vi "KE6221 -- Set Sine Wave Params.vi"(0 "Resource In":refnum<visa-resource-name>, 1 "Check For SCPI Errors? (T)":bool=TRUE, 7 "Sine Wave Params In":T1={"Frequency (Hz)"=1000.0, "Amplitude (A)"=0.001, "Offset (A)"=0.0, "Ranging Mode"=enum."Best", "Fixed Range"=enum."2mA", "Playback Mode"=enum."Time", "Time (s)"=1.0, "Num Cycles"=1.0, "Phase\nMarker?"=FALSE, "Phase Marker (deg)"=180.0, "Trig Link Line"=enum."1"} {"Offset (A)" min=-0.105 max=0.105 format="%.4p"; "Num Cycles" min=0.001 max=99999999900.0 format="%.3p"; "Time (s)" min=1e-07 max=999999.999 format="%.3p"; "Phase Marker (deg)" min=0.0 max=360.0 format="%.3f"; "Amplitude (A)" min=2e-12 max=0.105 format="%.3p"; "Frequency (Hz)" min=0.001 max=100000.0 format="%.3p"}, 11 "error in (no error)":errorcluster, 12 "Read Back Set Values? (T)":bool=TRUE) -> (4 "Resource Out (dupl)":refnum<visa-resource-name>, 8 "Sine Wave Params Out":T1={"Frequency (Hz)"=1000.0, "Amplitude (A)"=0.001, "Offset (A)"=0.0, "Ranging Mode"=enum."Best", "Fixed Range"=enum."2mA", "Playback Mode"=enum."Time", "Time (s)"=1.0, "Num Cycles"=1.0, "Phase\nMarker?"=FALSE, "Phase Marker (deg)"=180.0, "Trig Link Line"=enum."1"} {"Offset (A)" min=-0.105 max=0.105 format="%.4p"; "Num Cycles" min=0.001 max=99999999900.0 format="%.3p"; "Time (s)" min=1e-07 max=999999.999 format="%.3p"; "Phase Marker (deg)" min=0.0 max=360.0 format="%.3f"; "Amplitude (A)" min=2e-12 max=0.105 format="%.3p"; "Frequency (Hz)" min=0.001 max=100000.0 format="%.3p"}, 15 "error out":errorcluster)   [LabVIEW 2019, in "Keithley 622x.lvlib"]
doc: "Sets the parameters for a sine wave. Note that this VI can only be used with the 6221, since the 6220 doesn't support this feature."
uses:
  Keithley 622x.lvlib
  Typedefs/KE6221 -- Wave Sine Wave Params.ctl
  Low Level/Typedefs/KE6221 -- Wave Frequency.ctl
  Low Level/Typedefs/KE6221 -- Wave Amplitude.ctl
  Source/Typedefs/KE622x -- Current Level.ctl
  Low Level/Typedefs/KE6221 -- Wave Ranging Mode.ctl
  Source/Typedefs/KE622x -- Current Ranges.ctl
  Low Level/Typedefs/KE6221 -- Wave Playback Mode.ctl
  Low Level/Typedefs/KE6221 -- Wave Playback Time.ctl
  Low Level/Typedefs/KE6221 -- Wave Playback Num Cycles.ctl
  Low Level/Typedefs/KE6221 -- Wave Phase Marker.ctl
  Trigger/Low Level/Typedefs/KE622x -- Trig Link Line.ctl
  Low Level/Typedefs/KE6221 -- Wave Type.ctl
  Source/Typedefs/KE622x -- Current Range.ctl
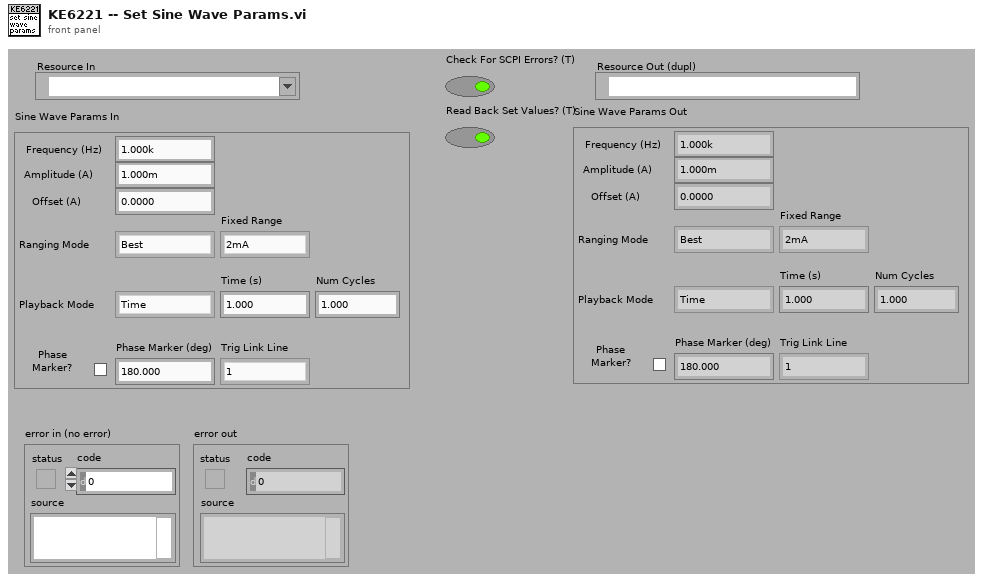
[diagram p1: front panel]
types:
  T1 = typedef "Keithley 622x.lvlib/KE6221 -- Wave Sine Wave Params.ctl" = cluster{"Frequency (Hz)":T2, "Amplitude (A)":T3, "Offset (A)":T4, "Ranging Mode":T5, "Fixed Range":T6, "Playback Mode":T7, "Time (s)":T8, "Num Cycles":T9, "Phase\nMarker?":bool, "Phase Marker (deg)":T10, "Trig Link Line":T11}
  T2 = typedef "Keithley 622x.lvlib/KE6221 -- Wave Frequency.ctl" = dbl
  T3 = typedef "Keithley 622x.lvlib/KE6221 -- Wave Amplitude.ctl" = dbl
  T4 = typedef "Keithley 622x.lvlib/KE622x -- Current Level.ctl" = dbl
  T5 = typedef "Keithley 622x.lvlib/KE6221 -- Wave Ranging Mode.ctl" = enum16{"Best", "Fixed"}
  T6 = typedef "Keithley 622x.lvlib/KE622x -- Current Ranges.ctl" = enum16{"2nA", "20nA", "200nA", "2uA", "20uA", "200uA", "2mA", "20mA", "100mA"}
  T7 = typedef "Keithley 622x.lvlib/KE6221 -- Wave Playback Mode.ctl" = enum16{"Time", "Num Cycles"}
  T8 = typedef "Keithley 622x.lvlib/KE6221 -- Wave Playback Time.ctl" = dbl
  T9 = typedef "Keithley 622x.lvlib/KE6221 -- Wave Playback Num Cycles.ctl" = dbl
  T10 = typedef "Keithley 622x.lvlib/KE6221 -- Wave Phase Marker.ctl" = dbl
  T11 = typedef "Keithley 622x.lvlib/KE622x -- Trig Link Line.ctl" = enum16{"1", "2", "3", "4", "5", "6"}
  T12 = typedef "Keithley 622x.lvlib/KE6221 -- Wave Type.ctl" = enum16{"Sinusoid", "Square", "Ramp", "Arbitrary 0", "Arbitrary 1", "Arbitrary 2", "Arbitrary 3", "Arbitrary 4"}
  T13 = typedef "Keithley 622x.lvlib/KE622x -- Current Range.ctl" = cluster{"Auto Range?":bool, "Man / Selected\nRange":T6}
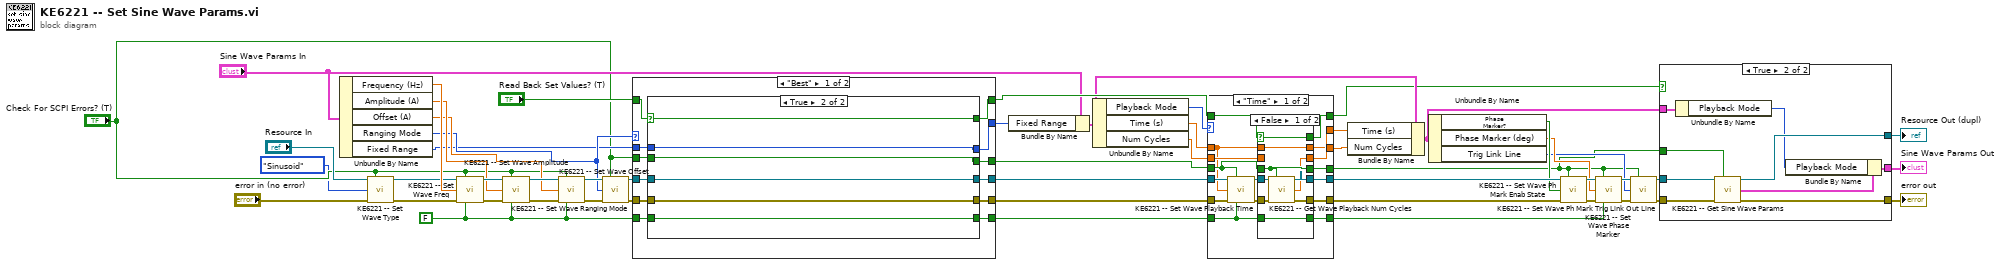
[diagram p0: block diagram]
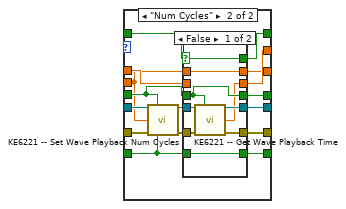
[diagram p4: hidden frame]
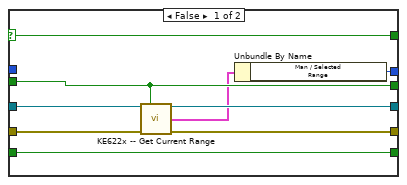
[diagram p6: hidden frame]
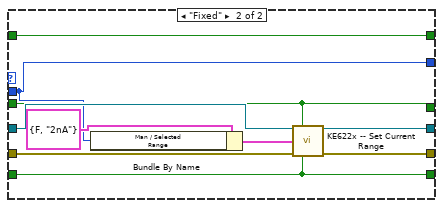
[diagram p7: hidden frame]
diagram:
  w17 = FALSE
  n1 = Unbundle By Name("Sine Wave Params In") -> ("Frequency (Hz)"=w40:T2, "Amplitude (A)"=w39:T3, "Offset (A)"=w38:T4, "Ranging Mode"=w37:T5, "Fixed Range"=w36:T6)
  n2 = call "KE6221 -- Set Wave Type.vi"("Resource In"="Resource In", "Check For SCPI Errors? (T)"="Check For SCPI Errors? (T)", "Wave Type"=KE6221_--_Wave_Type."Sinusoid", "error in (no error)"="error in (no error)") -> ("Resource Out (dupl)"=w8:refnum<visa-resource-name>, "error out"=w7:errorcluster)  [unwired: 10 in]
  n3 = call "KE6221 -- Set Wave Freq.vi"("Resource In"=w8, "Check For SCPI Errors? (T)"="Check For SCPI Errors? (T)", "Wave Frequency In (Hz)"=w40, "error in (no error)"=w7, "Read Back Set Value? (T)"=w17) -> ("Resource Out (dupl)"=w52:refnum<visa-resource-name>, "error out"=w51:errorcluster)  [unwired: 8 in, 1 out]
  n4 = call "KE6221 -- Set Wave Amplitude.vi"("Resource In"=w52, "Check For SCPI Errors? (T)"="Check For SCPI Errors? (T)", "Wave Amplitude In"=w39, "error in (no error)"=w51, "Read Back Set Value? (T)"=w17) -> ("Resource Out (dupl)"=w48:refnum<visa-resource-name>, "error out"=w47:errorcluster)  [unwired: 8 in, 1 out]
  n5 = call "KE6221 -- Set Wave Offset.vi"("Resource In"=w48, "Check For SCPI Errors? (T)"="Check For SCPI Errors? (T)", "Wave Offset In (A)"=w38, "error in (no error)"=w47, "Read Back Set Value? (T)"=w17) -> ("Resource Out (dupl)"=w46:refnum<visa-resource-name>, "error out"=w45:errorcluster)  [unwired: 8 in, 1 out]
  n6 = call "KE6221 -- Set Wave Ranging Mode.vi"("Resource In"=w46, "Check For SCPI Errors? (T)"="Check For SCPI Errors? (T)", "Ranging Mode"=w37, "error in (no error)"=w45) -> ("Resource Out (dupl)"=w50:refnum<visa-resource-name>, "error out"=w49:errorcluster)  [unwired: 10 in]
  n7 = case shown="\"Best\"" w37 {
    tunnel: w50 -> [w63 w89]
    tunnel: w49 -> [w62 w88]
    tunnel: [w59 w87] -> w33
    tunnel: [w60 w86] -> w30
    tunnel: "Check For SCPI Errors? (T)" -> [w61 w82]
    tunnel: w36 -> [w56 w81]
    tunnel: "Read Back Set Values? (T)" -> [w64 w83]
    tunnel: [w58 w82] -> w29
    tunnel: [w57 w83] -> w28
    tunnel: [w55 w81] -> w26
    tunnel: w17 -> [w54 w80]
    tunnel: [w53 w80] -> w16
    frame "Best" {
      n8 = case shown="True" w64 {
        selector: w64 -> [w68 w79]
        tunnel: w63 -> [w73 w77]
        tunnel: w62 -> [w72 w76]
        tunnel: w61 -> [w69 w78]
        tunnel: [w71 w76] -> w60
        tunnel: [w70 w77] -> w59
        tunnel: [w69 w78] -> w58
        tunnel: [w68 w79] -> w57
        tunnel: w56 -> [_ w75]
        tunnel: [w66 w75] -> w55
        tunnel: w54 -> [w65 w74]
        tunnel: [w65 w74] -> w53
        frame False {
          n9 = call "KE622x -- Get Current Range.vi"("Resource In"=w73, "Check For SCPI Errors? (T)"=w69, "error in (no error)"=w72) -> ("Resource Out (dupl)"=w70:refnum<visa-resource-name>, "Current Range"=w67:T13, "error out"=w71:errorcluster)  [unwired: 10 in]
          n10 = Unbundle By Name(w67) -> ("Man / Selected\nRange"=w66:T6)
        }
        frame True {
        }
      }
    }
    frame "Fixed" {
      n11 = Bundle By Name(cluster=T13 {"Auto Range?"=FALSE, "Man / Selected\nRange"=enum."2nA"} ("Current Range In"), "Man / Selected\nRange"=w81) -> (w84:T13)
      n12 = call "KE622x -- Set Current Range.vi"("Resource In"=w89, "Check For SCPI Errors? (T)"=w82, "Current Range In"=w84, "error in (no error)"=w88, "Read Back Set Values? (T)"=w80) -> ("Resource Out (dupl)"=w87:refnum<visa-resource-name>, "error out"=w86:errorcluster)  [unwired: 8 in, 1 out]
    }
  }
  n13 = Bundle By Name(cluster="Sine Wave Params In", "Fixed Range"=w26) -> (w25:T1)
  n14 = Unbundle By Name(w25) -> ("Playback Mode"=w34:T7, "Time (s)"=w32:T8, "Num Cycles"=w31:T9)
  n15 = case shown="\"Time\"" w34 {
    tunnel: w33 -> [w105 w137]
    tunnel: w32 -> [w94 w128]
    tunnel: w31 -> [w96 w126]
    tunnel: w30 -> [w104 w136]
    tunnel: w29 -> [w100 w132]
    tunnel: w28 -> [w103 w135]
    tunnel: [w95 w125] -> w23
    tunnel: [w99 w131] -> w11
    tunnel: [w98 w130] -> w22
    tunnel: [w97 w129] -> w21
    tunnel: [w93 w127] -> w24
    tunnel: w16 -> [w92 w124]
    tunnel: [w91 w123] -> w15
    tunnel: [w90 w122] -> w14
    frame "Time" {
      n16 = call "KE6221 -- Set Wave Playback Time.vi"("Resource In"=w105, "Check For SCPI Errors? (T)"=w100, "Playback Time (s) In"=w94, "error in (no error)"=w104, "Read Back Set Value? (T)"=w92) -> ("Resource Out (dupl)"=w102:refnum<visa-resource-name>, "error out"=w101:errorcluster)  [unwired: 8 in, 1 out]
      n17 = case shown="False" w103 {
        selector: w103 -> [w106 w115]
        tunnel: w102 -> [w114 w119]
        tunnel: w101 -> [w113 w120]
        tunnel: w100 -> [w112 w121]
        tunnel: [w112 w121] -> w99
        tunnel: [w111 w120] -> w97
        tunnel: [w110 w119] -> w98
        tunnel: w96 -> [_ w118]
        tunnel: [w109 w118] -> w95
        tunnel: w94 -> [w108 w117]
        tunnel: [w108 w117] -> w93
        tunnel: w92 -> [w107 w116]
        tunnel: [w107 w116] -> w91
        tunnel: [w106 w115] -> w90
        frame False {
          n18 = call "KE6221 -- Get Wave Playback Num Cycles.vi"("Resource In"=w114, "Check For SCPI Errors? (T)"=w112, "error in (no error)"=w113) -> ("Resource Out (dupl)"=w110:refnum<visa-resource-name>, "Num Cycles"=w109:T9, "error out"=w111:errorcluster)  [unwired: 10 in]
        }
        frame True {
        }
      }
    }
    frame "Num Cycles" {
      n19 = call "KE6221 -- Set Wave Playback Num Cycles.vi"("Resource In"=w137, "Check For SCPI Errors? (T)"=w132, "Num Cycles In"=w126, "error in (no error)"=w136, "Read Back Set Value? (T)"=w124) -> ("Resource Out (dupl)"=w134:refnum<visa-resource-name>, "error out"=w133:errorcluster)  [unwired: 8 in, 1 out]
      n20 = case shown="False" w135 {
        selector: w135 -> [w138 w147]
        tunnel: w134 -> [w146 w151]
        tunnel: w133 -> [w145 w152]
        tunnel: w132 -> [w144 w153]
        tunnel: [w144 w153] -> w131
        tunnel: [w143 w152] -> w129
        tunnel: [w142 w151] -> w130
        tunnel: w128 -> [_ w150]
        tunnel: [w141 w150] -> w127
        tunnel: w126 -> [w140 w149]
        tunnel: [w140 w149] -> w125
        tunnel: w124 -> [w139 w148]
        tunnel: [w139 w148] -> w123
        tunnel: [w138 w147] -> w122
        frame False {
          n21 = call "KE6221 -- Get Wave Playback Time.vi"("Resource In"=w146, "Check For SCPI Errors? (T)"=w144, "error in (no error)"=w145) -> ("Resource Out (dupl)"=w142:refnum<visa-resource-name>, "Playback Time (s)"=w141:T8, "error out"=w143:errorcluster)  [unwired: 10 in]
        }
        frame True {
        }
      }
    }
  }
  n22 = Bundle By Name(cluster=w25, "Time (s)"=w24, "Num Cycles"=w23) -> (w10:T1)
  n23 = Unbundle By Name(w10) -> ("Phase\nMarker?"=w20:bool, "Phase Marker (deg)"=w19:T10, "Trig Link Line"=w18:T11)
  n24 = call "KE6221 -- Set Wave Ph Mark Enab State.vi"("Resource In"=w22, "Check For SCPI Errors? (T)"=w11, "Phase Marker Enabled?"=w20, "error in (no error)"=w21) -> ("Resource Out (dupl)"=w44:refnum<visa-resource-name>, "error out"=w43:errorcluster)  [unwired: 10 in]
  n25 = call "KE6221 -- Set Wave Phase Marker.vi"("Resource In"=w44, "Check For SCPI Errors? (T)"=w11, "Phase Marker In (deg)"=w19, "error in (no error)"=w43, "Read Back Set Value? (T)"=w15) -> ("Resource Out (dupl)"=w42:refnum<visa-resource-name>, "error out"=w41:errorcluster)  [unwired: 8 in, 1 out]
  n26 = call "KE6221 -- Set Wave Ph Mark Trig Link Out Line.vi"("Resource In"=w42, "Check For SCPI Errors? (T)"=w11, "Trig Link Out Line"=w18, "error in (no error)"=w41) -> ("Resource Out (dupl)"=w13:refnum<visa-resource-name>, "error out"=w12:errorcluster)  [unwired: 10 in]
  n27 = case shown="True" w14 {
    tunnel: w13 -> [w155 w165]
    tunnel: w12 -> [w154 w164]
    tunnel: w11 -> [_ w163]
    tunnel: [w155 w162] -> w2
    tunnel: [w154 w161] -> w1
    tunnel: w10 -> [w156 w160]
    tunnel: [w156 w157] -> w9
    frame False {
    }
    frame True {
      n28 = Unbundle By Name(w160) -> ("Playback Mode"=w158:T7)
      n29 = call "KE6221 -- Get Sine Wave Params.vi"("Resource In"=w165, "Check For SCPI Errors? (T)"=w163, "error in (no error)"=w164) -> ("Resource Out (dupl)"=w162:refnum<visa-resource-name>, "Sine Wave Params"=w159:T1, "error out"=w161:errorcluster)  [unwired: 10 in]
      n30 = Bundle By Name(cluster=w159, "Playback Mode"=w158) -> (w157:T1)
    }
  }
  "Resource Out (dupl)" <- w2
  "error out" <- w1
  "Sine Wave Params Out" <- w9
